vi "Curtin_MouseBusy.vi"(7 "VI in":refnum<vi>, 9 "element":string, 11 "queue in":refnum<queue>) -> (3 "queue out":refnum<queue>)   [LabVIEW 2022 SP3]
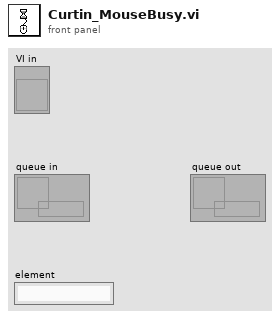
[diagram p1: front panel]
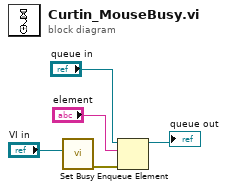
[diagram p0: block diagram]
diagram:
  n1 = call <vilib>:"Set Busy.vi"("VI reference (current VI)"="VI in") -> ("error out"=w4:errorcluster)  [unwired: 9 in, 1 out]
  n2 = Enqueue Element(queue="queue in", element="element", error in (no error)=w4) -> (queue out=→"queue out":refnum<queue>)  [unwired: 1 in, 2 out]
